vi "N_max_forsed_bitB.vi"(3 "On":bool[](array[boolean])) -> (0 "N":i32)   [LabVIEW 2019]
uses:
  Logik.lvlib
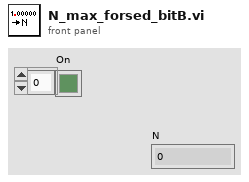
[diagram p1: front panel]
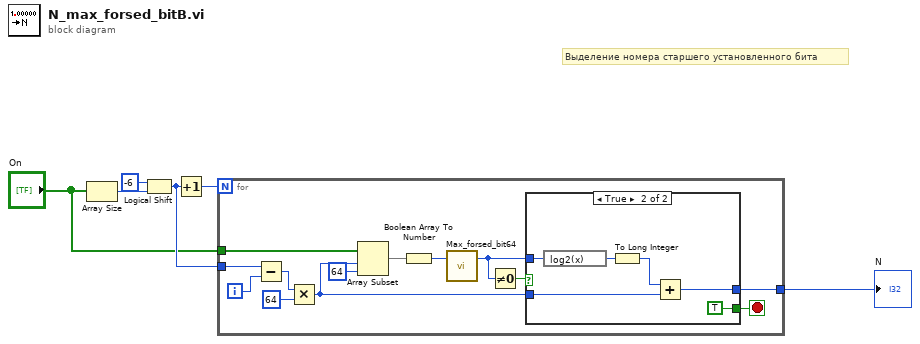
[diagram p0: block diagram]
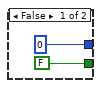
[diagram p2: hidden frame]
diagram:
  # "Выделение номера старшего установленного бита"
  n1 = Array Size(array="On") -> (size(s)=w6:i32)
  n2 = Logical Shift(y=i16 -6, x=w6) -> (x << y=w3:i32)
  n3 = Increment(x=w3) -> (x+1=w4:i32)
  n4 = for {
    N: w4 -> [_]
    tunnel: "On" -> [w17]
    tunnel: [w10] -> w2
    tunnel: w3 -> [w9]
    i -> [w8]
    stop <- w11 stop-if-true
    n5 = Subtract(x=w9, y=w8) -> (x-y=w7:i32)
    n6 = Multiply(x=w7, y=64 ("length")) -> (x*y=w12:i32)
    n7 = Array Subset(array=w17, index=w12, length=64) -> (w19:bool[])
    n8 = Boolean Array To Number(Boolean array=w19) -> (number=w15:u64)
    n9 = call "Max_forsed_bit64.vi"("IN"=w15) -> ("N"=w13:u64)  [unwired: 2 in]
    n10 = Not Equal To 0?(x=w13) -> (x != 0?=w14:bool)
    n11 = case shown="True" w14 {
      tunnel: w13 -> [_ w23]
      tunnel: w12 -> [_ w27]
      tunnel: [FALSE ("new element/subarray") TRUE ("new element/subarray")] -> w11
      tunnel: [0 w26] -> w10
      frame False {
      }
      frame True {
        n12 = expression code="log2(x)"(w23) -> (w22:u64)
        n13 = To Long Integer(number=w22) -> (32bit integer=w24:i32)
        n14 = Add(x=w24, y=w27) -> (x+y=w26:i32)
      }
    }
  }
  "N" <- w2
